vi "Koheras_get_set_Status.vi"(8 "error in":errorcluster, 9 "Array 2":i32[](array[numeric]), 10 "Array":string[](array[string]), 11 "VISA resource name in":refnum<visa-resource-name>) -> (0 "error out":errorcluster, 2 "Return":string[](array[string]), 3 "VISA resource name out":refnum<visa-resource-name>)   [LabVIEW 2013]
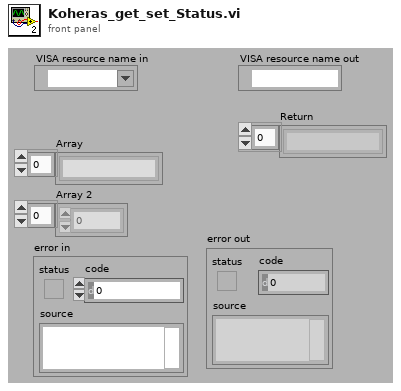
[diagram p1: front panel]
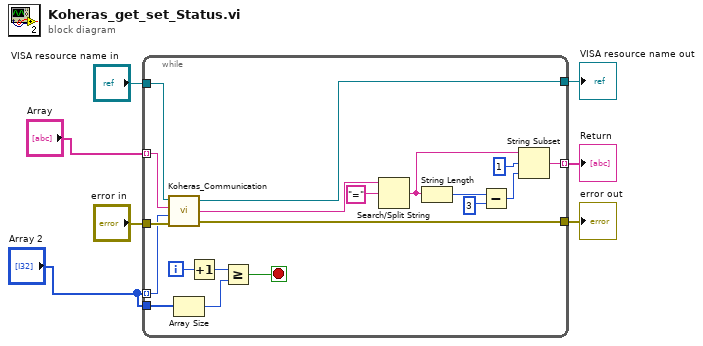
[diagram p0: block diagram]
diagram:
  n1 = while {
    tunnel: [w19] -> w3 mode=indexing
    tunnel: "error in" -> [w18]
    tunnel: "VISA resource name in" -> [w17]
    tunnel: [w16] -> w5
    tunnel: [w15] -> w4
    tunnel: "Array 2" -> [w12] mode=indexing
    tunnel: "Array" -> [w13] mode=indexing
    tunnel: "Array 2" -> [w11]
    i -> [w9]
    stop <- w14 stop-if-true
    n2 = call "Koheras_Communication.vi"("Error in"=w18, "Answer length"=w12, "Command"=w13, "VISA resource name in"=w17) -> ("Error out"=w15:errorcluster, "Returns"=w26:string, "VISA resource name out"=w16:refnum<visa-resource-name>)
    n3 = Array Size(array=w11) -> (size(s)=w10:i32)
    n4 = Increment(x=w9) -> (x+1=w8:i32)
    n5 = Greater Or Equal?(x=w8, y=w10) -> (x >= y?=w14:bool)
    n6 = Search/Split String(string=w26, search string/char (-)="=") -> (match + rest of string=w21:string)  [unwired: 3 out]
    n7 = String Length(string=w21) -> (length=w22:i32)
    n8 = Subtract(x=w22, y=3) -> (x-y=w24:i32)
    n9 = String Subset(string=w21, offset (0)=1, length (rest)=w24) -> (substring=w19:string)
  }
  "Return" <- w3
  "VISA resource name out" <- w5
  "error out" <- w4
